vi "Unflatten UIP Value.vi"(10 "String Value":string, 11 "ValueUIP In":refnum<class "ValueUIP.lvclass">) -> (0 "Error Out":errorcluster, 3 "ValueUIP Out":refnum<class "ValueUIP.lvclass">)   [LabVIEW 2020, in "UIM.lvlib" / "ValueUIP.lvclass"]
doc: "Overwrite this abstract method to implement child behavior for unflattening the UIP private data from XML compatible string format."
uses:
  ValueUIP.lvclass
  ValueUIP.lvclass/ValueUIP.ctl
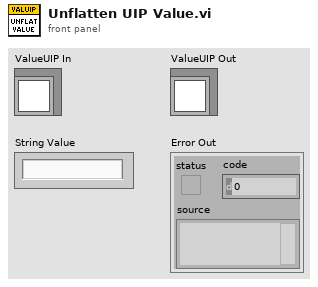
[diagram p1: front panel]
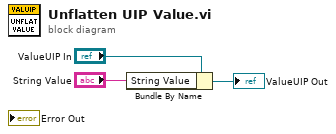
[diagram p0: block diagram]
diagram:
  n1 = Bundle By Name(cluster="ValueUIP In", "String Value"="String Value") -> (→"ValueUIP Out":refnum<class "ValueUIP.lvclass">)
